vi "Read DHT11.vi"(0 "LINX In":T1, 1 "Error In":errorcluster) -> (2 "LINX Out":T1, 3 "Relative Humidity":u8, 4 "Temperature (C)":u8, 5 "Error Out":errorcluster)   [LabVIEW 2020]
uses:
  <vilib>/MakerHub/LINX/Private/Type Defs/LINX Ref.ctl
  <vilib>/MakerHub/LINX/Private/Type Defs/Platform.ctl
  <vilib>/MakerHub/LINX/Private/Type Defs/Interface.ctl
  <vilib>/MakerHub/LINX/Private/Device/Type Defs/LINX Device Config.ctl
  <vilib>/MakerHub/LINX/Private/Device/Type Defs/TCP Config.ctl
  <vilib>/MakerHub/LINX/Private/Device/Type Defs/Channels.ctl
  <vilib>/MakerHub/LINX/LMH-LINX.lvlib
  <vilib>/MakerHub/LINX/Private/Device/Device.lvlib
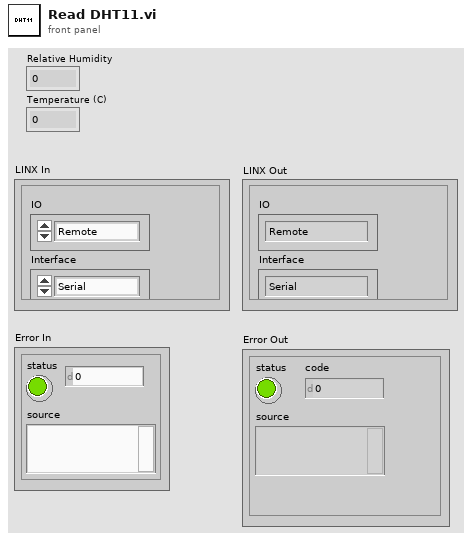
[diagram p1: front panel]
types:
  T1 = typedef "LMH-LINX.lvlib/LINX Ref.ctl" = cluster{"IO":T2, "Interface":T3, "LINX Device Config":T4}
  T2 = typedef "LMH-LINX.lvlib/Platform.ctl" = enum16{"Remote", "Local"}
  T3 = typedef "LMH-LINX.lvlib/Interface.ctl" = enum16{"Serial", "TCP"}
  T4 = typedef "LMH-LINX.lvlib/Device.lvlib/LINX Device Config.ctl" = cluster{"Interface":T3, "COM Port":refnum<visa-resource-name>, "TCP Configuration":T5, "Device Family":u8, "Device ID":u8, "Device Name":string, "TCP Ref":refnum<k5>, "Channels":T6}
  T5 = typedef "LMH-LINX.lvlib/Device.lvlib/TCP Config.ctl" = cluster{"IP Address":string, "Port":u16}
  T6 = typedef "LMH-LINX.lvlib/Channels.ctl" = cluster{"DI":u8[], "DO":u8[], "AI":u8[], "AO":u8[], "PWM":u8[], "QE":u8[], "UART":u8[], "I2C 2":u8[], "SPI":u8[], "CAN":u8[], "Servo":u8[], "AI Ref (V)":dbl, "AI Resolution (Bits)":u8, "AO Ref (V)":dbl, "AO Resolution (Bits)":u8}
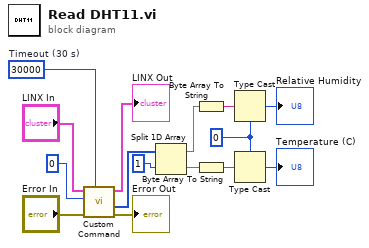
[diagram p0: block diagram]
diagram:
  w9 = u8 0
  w6 = 30000  # Timeout (30 s)
  n1 = call <vilib>:"Custom Command.vi"("Timeout (100 ms)"=w6, "Error In"="Error In", "Custom Command Number"=u16 0, "LINX Resource"="LINX In") -> ("Error Out"=→"Error Out":errorcluster, "Response"=w13:u8[], "LINX Resource"=→"LINX Out":T1)  [unwired: 4 in, 1 out]
  n2 = Split 1D Array(array=w13, index=1) -> (first subarray=w11:u8[], second subarray=w10:u8[])
  n3 = Byte Array To String(unsigned byte array=w11) -> (string=w15:string)
  n4 = Byte Array To String(unsigned byte array=w10) -> (string=w14:string)
  n5 = Type Cast(type=w9, x=w15) -> (*(type *) &x=→"Relative Humidity":u8)
  n6 = Type Cast(type=w9, x=w14) -> (*(type *) &x=→"Temperature (C)":u8)
